vi "9219_Thermocouple_Raw_to_Temp.vi"(9 "ThermocoupleType":u16(ring)=6 items=["B", "E", "J", "K", "R", "S", "T", "N"], 10 "CJC0":u32, 11 "Temp0":i32) -> (3 "T":dbl)   [LabVIEW 2019]
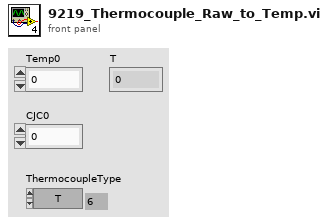
[diagram p1: front panel]
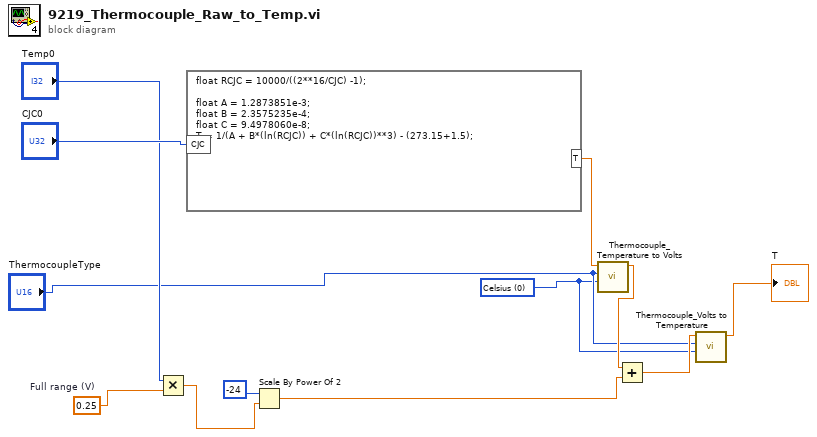
[diagram p0: block diagram]
diagram:
  w2 = u16 0 items=["Celsius", "Fahrenheit", "Kelvin", "Rankine"] ("Temperature Units")
  w10 = 0.25  # Full range (V)
  n1 = Multiply(x="Temp0", y=w10) -> (x*y=w9:dbl)
  n2 = formula code="float RCJC = 10000/((2**16/CJC) -1);\n\nfloat A = 1.2873851e-3;\nfloat B = 2.3575235e-4;\nfloat C = 9.4978060e-8;\nT = 1/(A + B*(ln(RCJC)) + C*(ln(RCJC))**3) - (273.15+1.5);"("CJC"="CJC0") -> ("T"=w7:dbl)
  n3 = Scale By Power Of 2(n=i16 -24, x=w9) -> (x*2^n=w5:dbl)
  n4 = call "Thermocouple_Temperature to Volts.vi"("Temperature Units"=w2, "ThermocoupleType"="ThermocoupleType", "Temperature"=w7) -> ("Thermocouple Voltage"=w6:sgl)  [unwired: 4 in]
  n5 = Add(x=w6, y=w5) -> (x+y=w4:dbl)
  n6 = call "Thermocouple_Volts to Temperature.vi"("Temperature Units"=w2, "ThermocoupleType"="ThermocoupleType", "Thermocouple Voltage"=w4) -> ("Temperature"=→"T":sgl)  [unwired: 4 in]
